vi "MH_WritePTURecordSgl.vi"(0 "refnum":refnum<file>, 2 "TTTR Records":u32, 3 "error in":errorcluster) -> (6 "refnum en sortie":refnum<file>, 10 "error out":errorcluster)   [LabVIEW 2019]
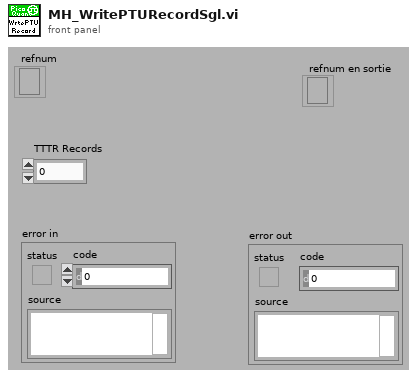
[diagram p1: front panel]
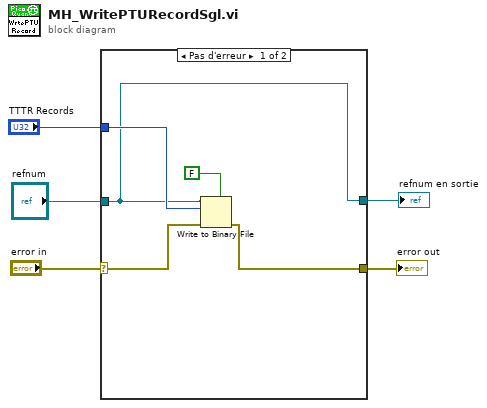
[diagram p0: block diagram]
diagram:
  n1 = case shown="Pas d'erreur" "error in" {
    selector: "error in" -> [w9 w12]
    tunnel: "refnum" -> [w7 w11]
    tunnel: [w10 w12] -> w4
    tunnel: "TTTR Records" -> [w8 _]
    tunnel: [w7 w11] -> w1
    frame No Error {
      n2 = Write to Binary File(file (use dialog)=w7, data=w8, error in=w9, 5:FALSE ("ajouter une taille de tableau ou de chaîne ? (V)")) -> (error out=w10:errorcluster)  [unwired: 2 in, 2 out]
    }
    frame Error {
    }
  }
  "error out" <- w4
  "refnum en sortie" <- w1
